vi "GetPackageVersionInfo_LV2015.vi"(8 "error in (no error)":errorcluster) -> (0 "error out":errorcluster, 3 "Package Version Info":string)   [LabVIEW 2015]
panel:
  # "Connector Pane"
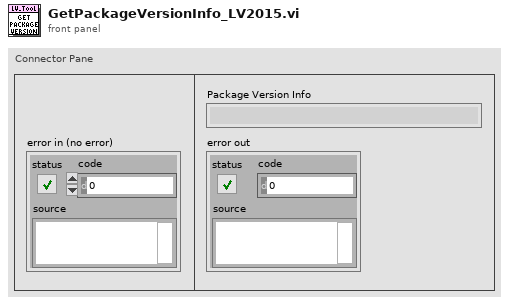
[diagram p1: front panel]
types:
  T1 = enum32{"invalid app kind", "Development System", "Run Time System", "Student Edition", "Embedded LabVIEW", "Evaluation", "Custom"}
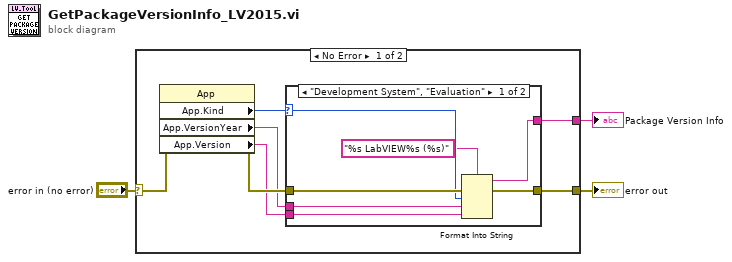
[diagram p0: block diagram]
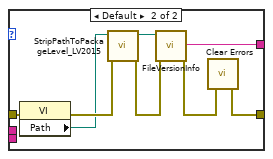
[diagram p2: hidden frame]
diagram:
  n1 = case shown="No Error" "error in (no error)" {
    selector: "error in (no error)" -> [w8 w26]
    tunnel: [w10 w26] -> w3
    tunnel: [w9 _] -> w2
    frame No Error {
      n2 = property class="App"(error in=w8) -> (error out=w7:errorcluster, "App.Kind"=w6:T1, "App.VersionYear"=w5:string, "App.Version"=w4:string)  [unwired: 1 in, 1 out]
      n3 = case shown="\"Development System\", \"Evaluation\"" w6 {
        selector: w6 -> [w15 _]
        tunnel: [w16 w25] -> w10
        tunnel: [w14 w24] -> w9
        tunnel: w7 -> [w17 w18]
        tunnel: w5 -> [w12 _]
        tunnel: w4 -> [w11 _]
        frame "Development System", "Evaluation" {
          n4 = Format Into String(format string="%s LabVIEW%s (%s)", error in=w17, w15, w12, w11) -> (resulting string=w14:string, error out=w16:errorcluster)  [unwired: 1 in]
        }
        frame Default {
          n5 = property class="VI"(error in=w18) -> (error out=w22:errorcluster, "Path"=w20:path)  [unwired: 1 in, 1 out]
          n6 = call "StripPathToPackageLevel_LV2015.vi"("error in (no error)"=w22, "Path in"=w20) -> ("error out"=w23:errorcluster, "Path out"=w21:path)  [unwired: 8 in]
          n7 = call <vilib>:"FileVersionInfo.vi"("error in (no error)"=w23, "Application Path in"=w21) -> ("error out"=w19:errorcluster, "File Version Info"=w24:string)  [unwired: 6 in, 2 out]
          n8 = call <vilib>:"Clear Errors.vi"("error in (no error)"=w19) -> ("error out"=w25:errorcluster)  [unwired: 5 in, 1 out]
        }
      }
    }
    frame Error {
    }
  }
  "error out" <- w3
  "Package Version Info" <- w2
